vi "TX.vi"() -> ()   [LabVIEW 2023]
uses:
  <vilib>/userDefined/High Color/IMAQdx.ctl
  TX_Cluster1TypeDef.ctl
  TX_Control 3.ctl
  TX_EnumTypeDef.ctl
  <vilib>/vision/Image Controls.llb/IMAQ Image.ctl
panel:
  in  "Select Camera:":T1
  in  "StartCam":bool
  out "CamView":T2(plugin-control)
  in  "EXIT":bool
  in  "Enable TCP":bool
  in  "Photo":bool
  in  "Stop":bool
  in  "START":bool
  in  "error in (no error) 2":errorcluster
  in  "error in (no error)":errorcluster
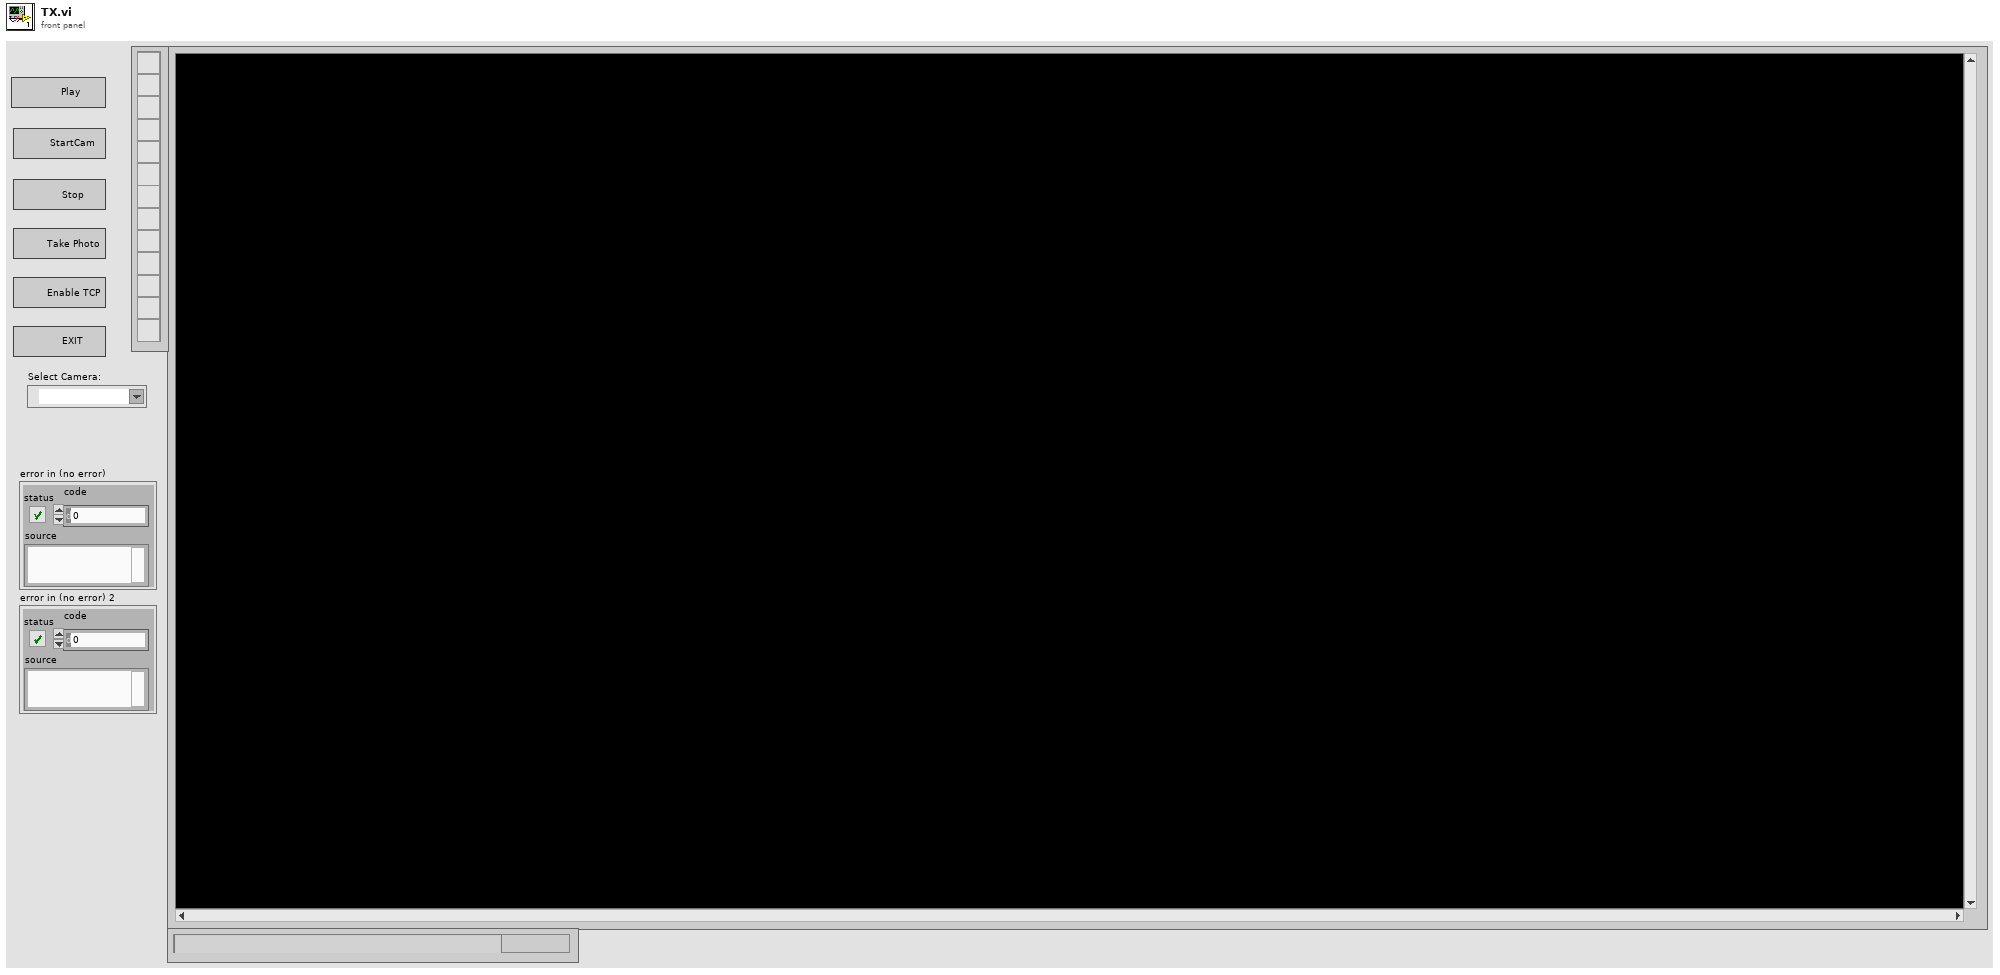
[diagram p1: front panel]
types:
  T1 = typedef "IMAQdx.ctl" = refnum<k21>
  T2 = typedef "IMAQ Image.ctl" = refnum<image>
  T3 = typedef "TX_EnumTypeDef.ctl" = enum16{"Initialize", "StartCam", "EnableTCP", "TakePhoto", "ShutDown"}
  T4 = cluster{"Enum":T3, "RawImage":T2, "Data":variant}
  T5 = typedef "TX_Control 3.ctl" = enum16{"Default", "StartCamera", "TakePhoto", "EnableTCP", "Cam2Display", "CloseAll"}
  T6 = cluster{"Enum":T5, "Data":variant, "Data2":variant}
  T7 = typedef "TX_Cluster1TypeDef.ctl" = cluster{"Enum":T5, "CamSel":variant, "CamView":variant}
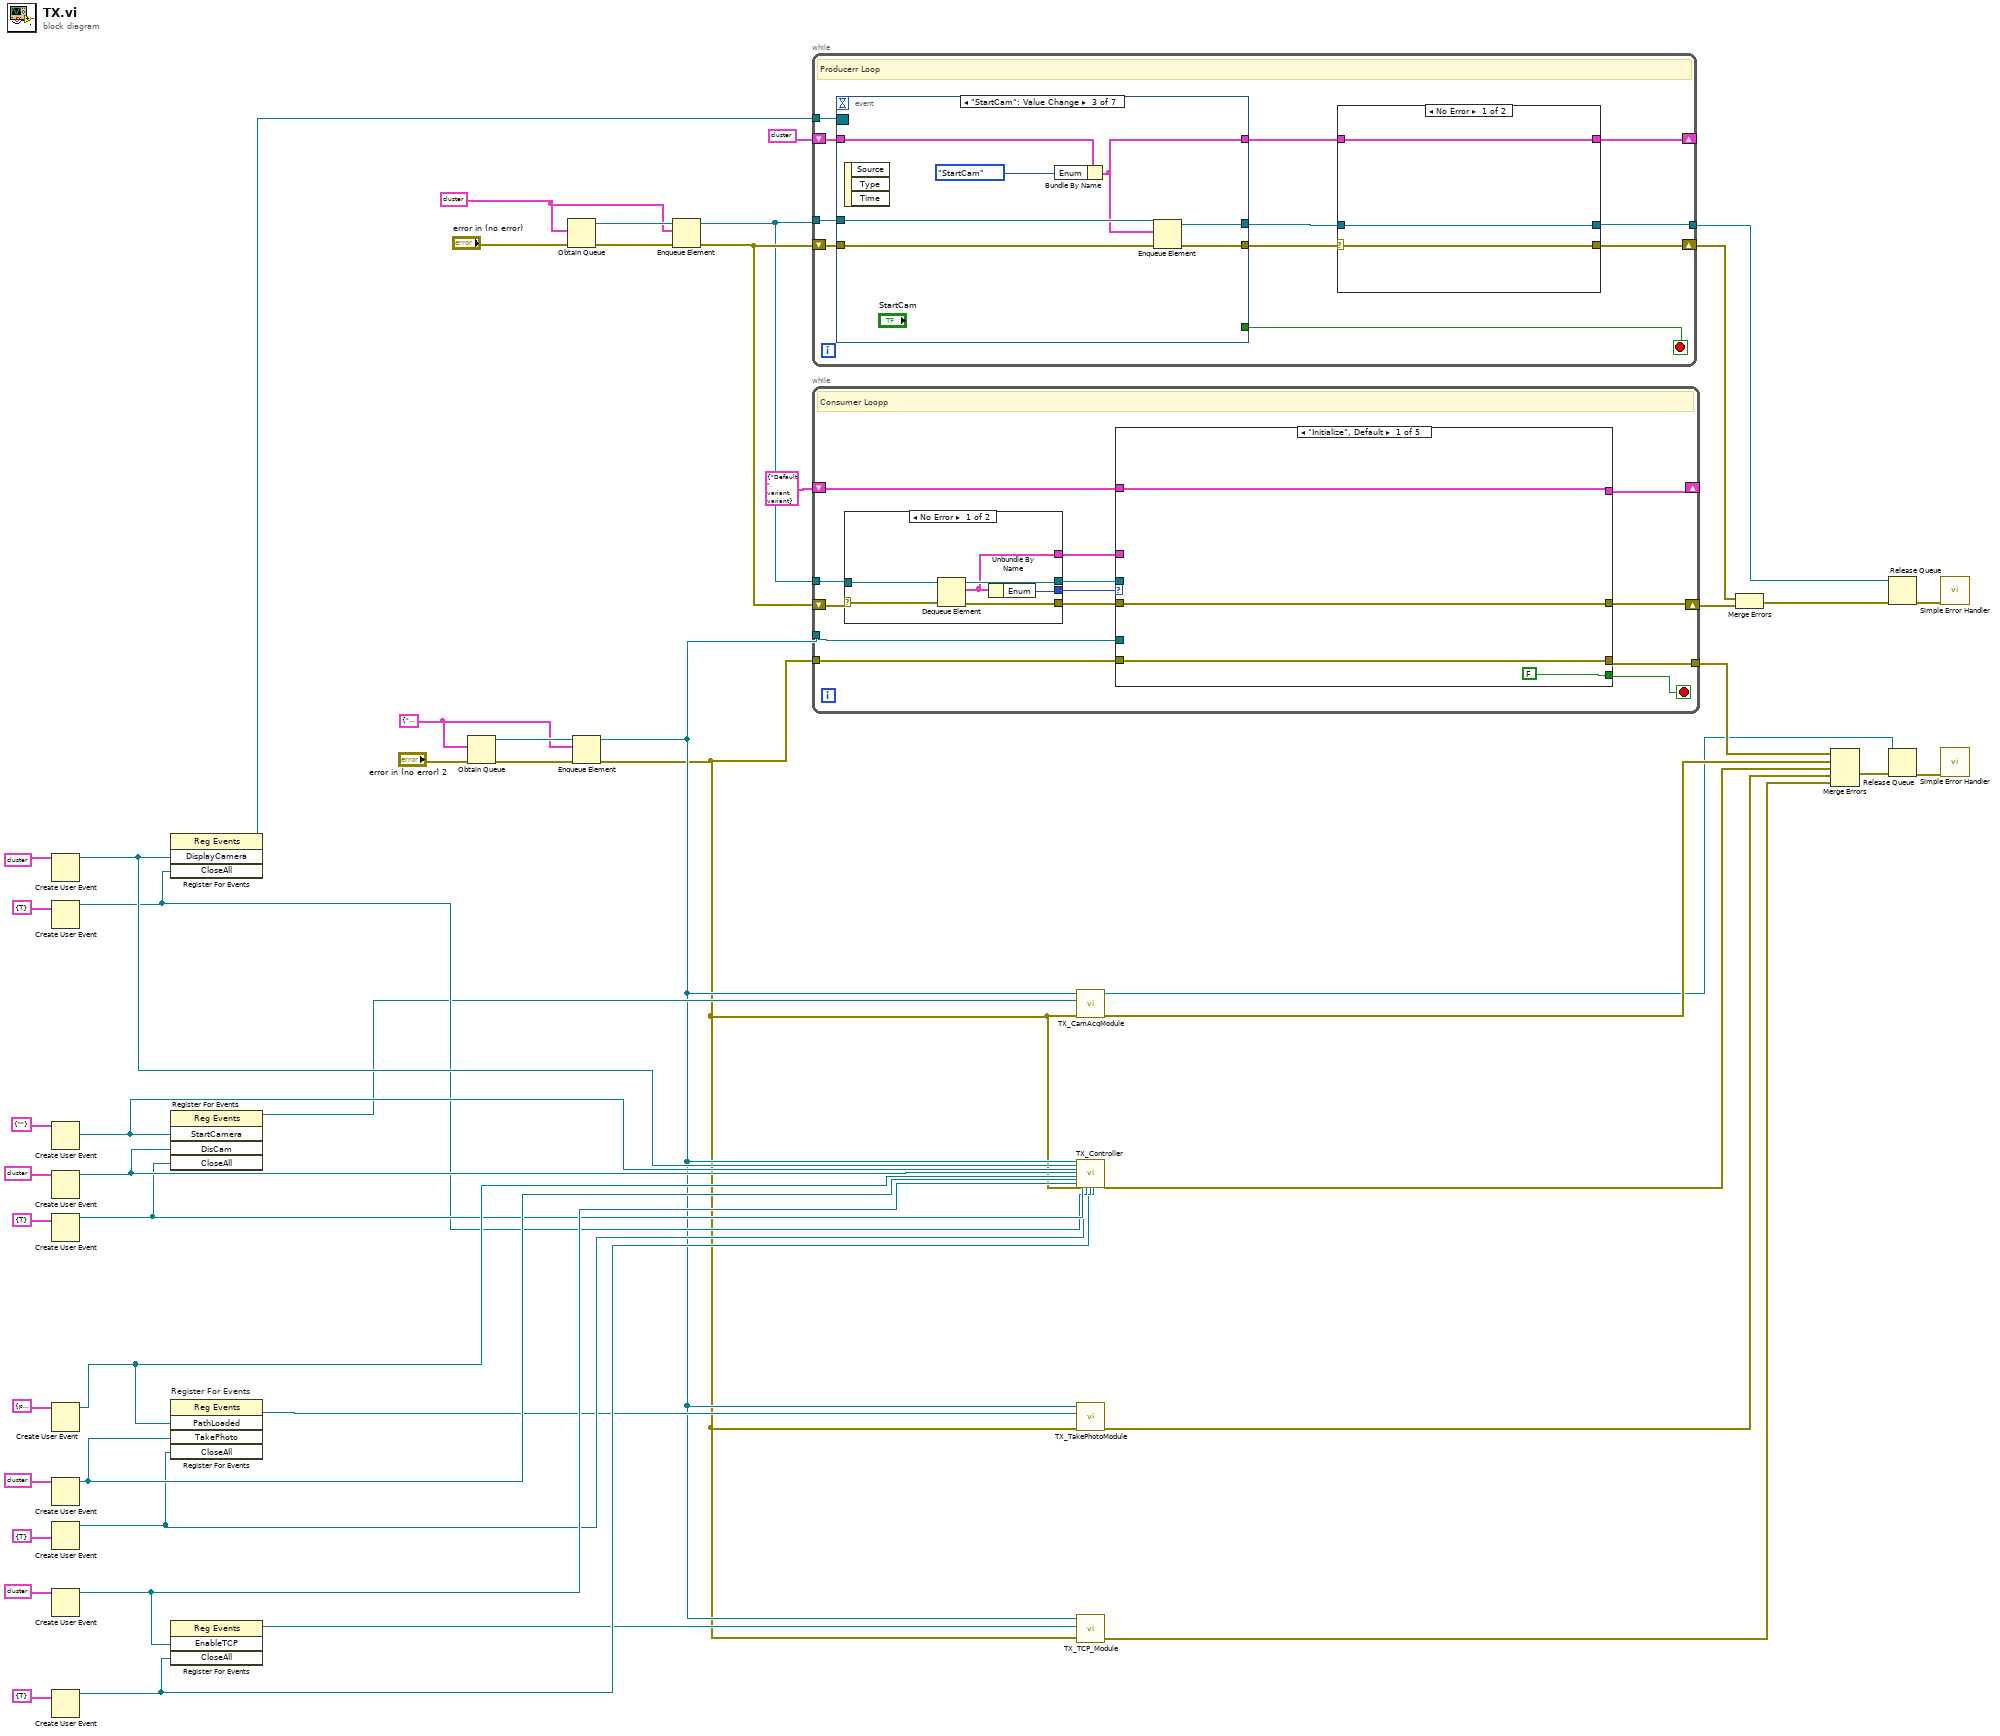
[diagram p0: block diagram]
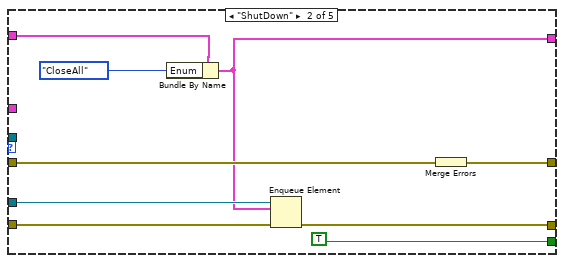
[diagram p2: hidden frame]
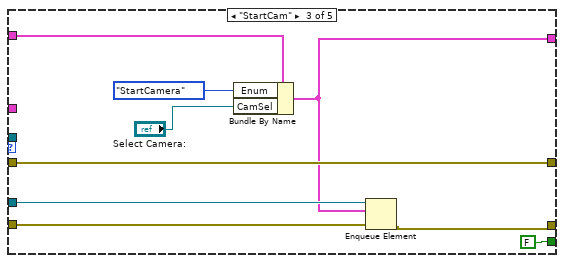
[diagram p3: hidden frame]
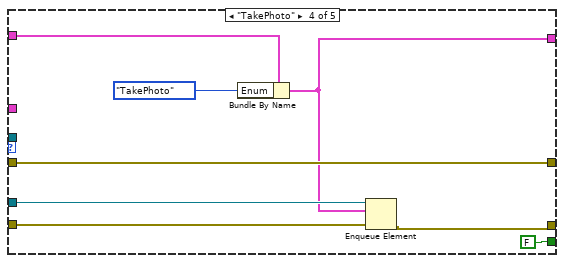
[diagram p4: hidden frame]
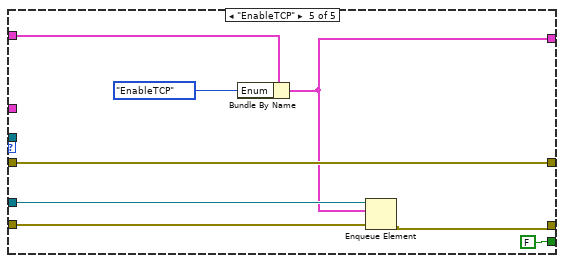
[diagram p5: hidden frame]
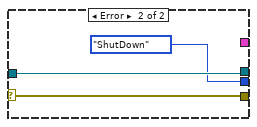
[diagram p6: hidden frame]
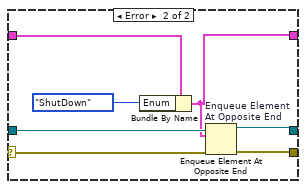
[diagram p7: hidden frame]
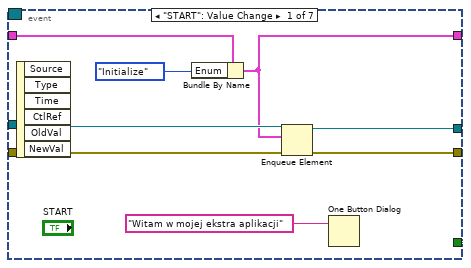
[diagram p8: hidden frame]
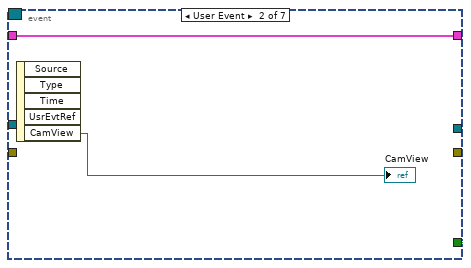
[diagram p9: hidden frame]
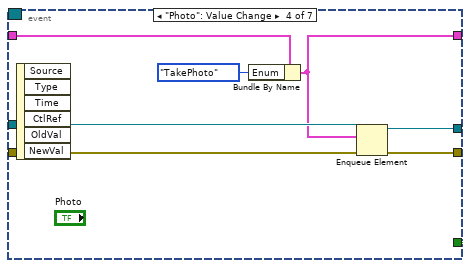
[diagram p10: hidden frame]
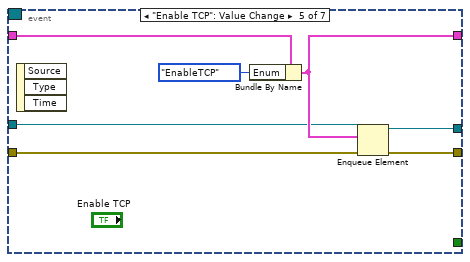
[diagram p11: hidden frame]
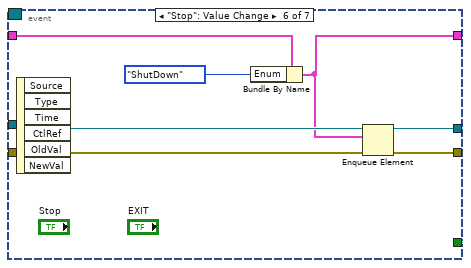
[diagram p12: hidden frame]
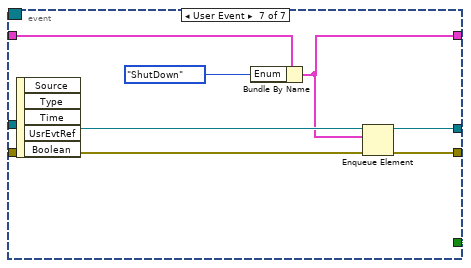
[diagram p13: hidden frame]
diagram:
  w32 = T4 {"Enum"=enum."Initialize", "RawImage"=refnum, "Data"=variant(refnum<image> refnum)} ("clusterSimple")
  w38 = T6 {"Enum"=enum."Default", "Data"=variant, "Data2"=variant(refnum<image> refnum)}
  n1 = Create User Event(user event datatype=cluster{"CamView":T2} {"CamView"=refnum} ("DisplayCamera")) -> (user event=w20:refnum<user-event>)  [unwired: 1 in, 1 out]
  n2 = Create User Event(user event datatype=cluster{"Boolean":bool} {"Boolean"=TRUE} ("CloseAll")) -> (user event=w13:refnum<user-event>)  [unwired: 1 in, 1 out]
  n3 = Create User Event(user event datatype=cluster{"CamSel":T1} {"CamSel"=""} ("StartCamera")) -> (user event=w19:refnum<user-event>)  [unwired: 1 in, 1 out]
  n4 = Create User Event(user event datatype=cluster{"CamView":T2} {"CamView"=refnum} ("DisCam")) -> (user event=w18:refnum<user-event>)  [unwired: 1 in, 1 out]
  n5 = Create User Event(user event datatype=cluster{"Boolean":bool} {"Boolean"=TRUE} ("CloseAll")) -> (user event=w14:refnum<user-event>)  [unwired: 1 in, 1 out]
  n6 = Create User Event(user event datatype=cluster{"File Path":path} {"File Path"=path ""} ("PathLoaded")) -> (user event=w17:refnum<user-event>)  [unwired: 1 in, 1 out]
  n7 = Create User Event(user event datatype=cluster{"CamView":T2} {"CamView"=refnum} ("TakePhoto")) -> (user event=w16:refnum<user-event>)  [unwired: 1 in, 1 out]
  n8 = Create User Event(user event datatype=cluster{"CloseAll":bool} {"CloseAll"=TRUE} ("CloseAll")) -> (user event=w12:refnum<user-event>)  [unwired: 1 in, 1 out]
  n9 = Create User Event(user event datatype=cluster{"CamView":T2} {"CamView"=refnum} ("EnableTCP")) -> (user event=w15:refnum<user-event>)  [unwired: 1 in, 1 out]
  n10 = Create User Event(user event datatype=cluster{"Boolean":bool} {"Boolean"=TRUE} ("CloseAll")) -> (user event=w11:refnum<user-event>)  [unwired: 1 in, 1 out]
  n11 = register-events(w20, w13) -> (reference out=w36:refnum<event-registration>)  [unwired: 2 in, 1 out]
  n12 = register-events(w19, w18, w14) -> (reference out=w4:refnum<event-registration>)  [unwired: 2 in, 1 out]
  n13 = register-events "Register For Events"(w17, w16, w12) -> (reference out=w9:refnum<event-registration>)  [unwired: 2 in, 1 out]
  n14 = register-events(w15, w11) -> (reference out=w7:refnum<event-registration>)  [unwired: 2 in, 1 out]
  n15 = Obtain Queue(element data type=w38, error in (no error)="error in (no error) 2") -> (queue out=w40:refnum<queue>, error out=w41:errorcluster)  [unwired: 3 in, 1 out]
  n16 = Obtain Queue(element data type=w32, error in (no error)="error in (no error)") -> (queue out=w50:refnum<queue>, error out=w51:errorcluster)  [unwired: 3 in, 1 out]
  n17 = Enqueue Element(queue=w40, element=w38, error in (no error)=w41) -> (queue out=w2:refnum<queue>, error out=w1:errorcluster)  [unwired: 1 in, 1 out]
  n18 = Enqueue Element(queue=w50, element=w32, error in (no error)=w51) -> (queue out=w47:refnum<queue>, error out=w48:errorcluster)  [unwired: 1 in, 1 out]
  n19 = while {
    shift-right: [w56] -> w46
    shift-left: w48 -> [w61]
    tunnel: w47 -> [w59]
    tunnel: [w57] -> w49
    tunnel: w36 -> [w55]
    shift-right: [w52] -> _
    shift-left: T4 {"Enum"=enum."Initialize", "RawImage"=refnum, "Data"=variant(refnum<image> refnum)} ("clusterSimple") -> [w54]
    stop <- w62 stop-if-true
    # "Producerr Loop"
    n20 = event shown="[2] \"StartCam\": Value Change" {
      selector: w55 -> [_ _ _ _ _ _ _]
      dyn-events: _ -> [_ _ _ _ _ _ _]
      timeout: _ -> [_ _ _ _ _ _ _]
      tunnel: [FALSE ("STOP") FALSE ("STOP") FALSE ("STOP") FALSE ("STOP") _ TRUE ("STOP") TRUE ("STOP")] -> w62
      tunnel: w61 -> [w80 _ w91 w99 w103 w115 w123]
      tunnel: [w79 _ w89 w97 w102 w114 w122] -> w60
      tunnel: w59 -> [w78 _ w92 w100 w104 w113 w121]
      tunnel: [w77 _ w90 w98 w101 w112 w120] -> w58
      tunnel: w54 -> [w76 w84 w88 w96 w105 w110 w118]
      tunnel: [w74 w84 w86 w95 w106 w108 w116] -> w53
      event "START": Value Change {
        n21 = event-data() -> ()  [unwired: 1 in, 6 out]
        n22 = Bundle By Name(cluster=w76, "Enum"=TX_EnumTypeDef."Initialize") -> (w74:T4)
        n23 = Enqueue Element(queue=w78, element=w74, error in (no error)=w80) -> (queue out=w77:refnum<queue>, error out=w79:errorcluster)  [unwired: 1 in, 1 out]
        n24 = One Button Dialog(message="Witam w mojej ekstra aplikacji") -> ()  [unwired: 1 in, 1 out]
      }
      event User Event {
        n25 = event-data() -> ("CamView"=→"CamView":T2)  [unwired: 1 in, 4 out]
      }
      event "StartCam": Value Change {
        n26 = event-data() -> ()  [unwired: 1 in, 3 out]
        n27 = Bundle By Name(cluster=w88, "Enum"=TX_EnumTypeDef."StartCam" ("element")) -> (w86:T4)
        n28 = Enqueue Element(queue=w92, element=w86, error in (no error)=w91) -> (queue out=w90:refnum<queue>, error out=w89:errorcluster)  [unwired: 1 in, 1 out]
      }
      event "Photo": Value Change {
        n29 = event-data() -> ()  [unwired: 1 in, 6 out]
        n30 = Bundle By Name(cluster=w96, "Enum"=TX_EnumTypeDef."TakePhoto") -> (w95:T4)
        n31 = Enqueue Element(queue=w100, element=w95, error in (no error)=w99) -> (queue out=w98:refnum<queue>, error out=w97:errorcluster)  [unwired: 1 in, 1 out]
      }
      event "Enable TCP": Value Change {
        n32 = event-data() -> ()  [unwired: 1 in, 3 out]
        n33 = Bundle By Name(cluster=w105, "Enum"=TX_EnumTypeDef."EnableTCP") -> (w106:T4)
        n34 = Enqueue Element(queue=w104, element=w106, error in (no error)=w103) -> (queue out=w101:refnum<queue>, error out=w102:errorcluster)  [unwired: 1 in, 1 out]
      }
      event "Stop": Value Change {
        n35 = event-data() -> ()  [unwired: 1 in, 6 out]
        n36 = Bundle By Name(cluster=w110, "Enum"=TX_EnumTypeDef."ShutDown") -> (w108:T4)
        n37 = Enqueue Element(queue=w113, element=w108, error in (no error)=w115) -> (queue out=w112:refnum<queue>, error out=w114:errorcluster)  [unwired: 1 in, 1 out]
      }
      event User Event {
        n38 = event-data() -> ()  [unwired: 1 in, 5 out]
        n39 = Bundle By Name(cluster=w118, "Enum"=TX_EnumTypeDef."ShutDown") -> (w116:T4)
        n40 = Enqueue Element(queue=w121, element=w116, error in (no error)=w123) -> (queue out=w120:refnum<queue>, error out=w122:errorcluster)  [unwired: 1 in, 1 out]
      }
    }
    n41 = case shown="No Error" w60 {
      selector: w60 -> [w64 w72]
      tunnel: [w65 w69] -> w57
      tunnel: w58 -> [w65 w70]
      tunnel: [w64 w71] -> w56
      tunnel: w53 -> [w63 w67]
      tunnel: [w63 w66] -> w52
      frame No Error {
      }
      frame Error {
        n42 = Bundle By Name(cluster=w67, "Enum"=TX_EnumTypeDef."ShutDown") -> (w66:T4)
        n43 = Enqueue Element At Opposite End "Enqueue Element \nAt Opposite End"(queue=w70, element=w66, error in (no error)=w72) -> (queue out=w69:refnum<queue>, error out=w71:errorcluster)  [unwired: 1 in, 1 out]
      }
    }
  }
  n44 = while {
    shift-right: [w132] -> w45
    shift-left: w48 -> [w136]
    tunnel: w47 -> [w135]
    tunnel: w2 -> [w130]
    tunnel: w1 -> [w129]
    tunnel: [w128] -> w34
    shift-right: [w126] -> _
    shift-left: T7 {"Enum"=enum."Default", "CamSel"=variant(refnum<image> refnum), "CamView"=variant(refnum<image> refnum)} ("Cluster") -> [w127]
    stop <- w124 stop-if-true
    # "Consumer Loopp"
    n45 = case shown="No Error" w136 {
      selector: w136 -> [w180 w183]
      tunnel: w135 -> [w178 w182]
      tunnel: [w179 w183] -> w133
      tunnel: [w177 w182] -> w131
      tunnel: [w176 TX_EnumTypeDef."ShutDown" ("Enum")] -> w134
      tunnel: [w175 _] -> w125
      frame No Error {
        n46 = Dequeue Element(queue=w178, error in (no error)=w180) -> (queue out=w177:refnum<queue>, element=w175:T4, error out=w179:errorcluster)  [unwired: 1 in, 1 out]
        n47 = Unbundle By Name(w175) -> ("Enum"=w176:T3)
      }
      frame Error {
      }
    }
    n48 = case shown="\"Initialize\", Default" w134 {
      tunnel: w133 -> [w140 w149 w153 w161 w169]
      tunnel: [w140 w148 w153 w161 w169] -> w132
      tunnel: w131 -> [_ _ _ _ _]
      tunnel: [FALSE TRUE FALSE FALSE FALSE] -> w124
      tunnel: w130 -> [_ w143 w158 w166 w174]
      tunnel: w129 -> [w137 w145 w157 w165 w173]
      tunnel: [w137 w144 w156 w164 w172] -> w128
      tunnel: w127 -> [w138 w146 w154 w162 w170]
      tunnel: [w138 w142 w151 w159 w167] -> w126
      tunnel: w125 -> [_ _ _ _ _]
      frame "Initialize", Default {
      }
      frame "ShutDown" {
        n49 = Bundle By Name(cluster=w146, "Enum"=TX_Control_3."CloseAll") -> (w142:T7)
        n50 = Enqueue Element(queue=w143, element=w142, error in (no error)=w145) -> (error out=w144:errorcluster)  [unwired: 1 in, 2 out]
        n51 = Merge Errors(w149) -> (w148:errorcluster)
      }
      frame "StartCam" {
        n52 = Bundle By Name(cluster=w154, "Enum"=TX_Control_3."StartCamera", "CamSel"="Select Camera:") -> (w151:T7)
        n53 = Enqueue Element(queue=w158, element=w151, error in (no error)=w157) -> (error out=w156:errorcluster)  [unwired: 1 in, 2 out]
      }
      frame "TakePhoto" {
        n54 = Bundle By Name(cluster=w162, "Enum"=TX_Control_3."TakePhoto") -> (w159:T7)
        n55 = Enqueue Element(queue=w166, element=w159, error in (no error)=w165) -> (error out=w164:errorcluster)  [unwired: 1 in, 2 out]
      }
      frame "EnableTCP" {
        n56 = Bundle By Name(cluster=w170, "Enum"=TX_Control_3."EnableTCP") -> (w167:T7)
        n57 = Enqueue Element(queue=w174, element=w167, error in (no error)=w173) -> (error out=w172:errorcluster)  [unwired: 1 in, 2 out]
      }
    }
  }
  n58 = call "TX_CamAcqModule.vi"("error out"=w1, "Event Registration Refnum"=w4, "queue out"=w2) -> ("error out 2"=w6:errorcluster, "queue out 2"=w5:refnum<queue>)  [unwired: 7 in]
  n59 = call "TX_Controller.vi"("queue out"=w2, "DisplayCamera"=w20, "StartCamera"=w19, "DisCam"=w18, "PathLoaded"=w17, "TakePhoto"=w16, "EnableTCP"=w15, "error out"=w1, "CloseAll"=w14, "CloseAll 2"=w13, "CloseAll 3"=w12, "CloseAll 4"=w11) -> ("error out 2"=w10:errorcluster)  [unwired: 15 in]
  n60 = call "TX_TakePhotoModule.vi"("error out"=w1, "Event Registration Refnum"=w9, "queue out"=w2) -> ("error out 2"=w8:errorcluster)  [unwired: 8 in]
  n61 = call "TX_TCP_Module.vi"("error out"=w1, "Event Registration Refnum"=w7, "queue out"=w2) -> ("error out 2"=w3:errorcluster)  [unwired: 8 in]
  n62 = Merge Errors(w46, w45) -> (w44:errorcluster)
  n63 = Merge Errors(w34, w6, w10, w8, w3) -> (w35:errorcluster)
  n64 = Release Queue(queue=w49, error in (no error)=w44) -> (error out=w42:errorcluster)  [unwired: 1 in, 2 out]
  n65 = Release Queue(queue=w5, error in (no error)=w35) -> (error out=w37:errorcluster)  [unwired: 1 in, 2 out]
  n66 = call <vilib>:"Simple Error Handler.vi"("error in (no error)"=w42) -> ()  [unwired: 4 in, 5 out]
  n67 = call <vilib>:"Simple Error Handler.vi"("error in (no error)"=w37) -> ()  [unwired: 4 in, 5 out]
